vi "Configure Digital Audio Task.vi"(8 "error in (no error)":errorcluster, 11 "digital generation":T2={"data channel list"="", "master clock channel list"="", "digital protocol settings"={"logic level"=enum."3.3 V", "PCM Data Configuration"={"Frame Sync Edge for Channel 0"=enum."Falling", "Channel Count Per Frame"=2, "Channel Length"=32, "Bit Depth"=24, "Channel 0 Offset"=1, "Endianness"=enum."MSB First", "Data Justification"=enum."Left Justified"}, "bit clock rate"=3025000.0, "master clock rate"=3025000.0, "clock mode"=enum."divided clock", "Frame Sync Clock Control"={"Frame Length"=64, "Frame Sync Pulse Width"=32, "Bit Clock Edge  Sync"=enum."Falling"}}, "signal settings"={"signal type"=enum."Sine", "properties"="", "output level units"=enum."% FS"}} {"digital protocol settings"."master clock rate" format="%.4p"; "digital protocol settings"."bit clock rate" format="%.4p"}) -> (0 "error out":errorcluster, 2 "master clock task":T1, 3 "data task":T1)   [LabVIEW 2021, in "DigitalAudioGenerationProcess.lvlib"]
uses:
  DigitalAudioGenerationProcess.lvlib
  controls/digital generation settings.ctl
  controls/digital protocol settings.ctl
  <vilib>/PDM Acquisition Toolkit/host/Classes/Session/Controls/Logic Levels.ctl
  <vilib>/PDM Acquisition Toolkit/shared/controls/PCM Data Format Configuration.ctl
  <vilib>/PDM Acquisition Toolkit/shared/controls/Digital Edge.ctl
  <vilib>/PDM Acquisition Toolkit/shared/controls/PCM Bit Endianness.ctl
  <vilib>/PDM Acquisition Toolkit/shared/controls/PCM Data Justification.ctl
  <vilib>/PDM Acquisition Toolkit/shared/controls/clock mode.ctl
  <vilib>/PDM Acquisition Toolkit/shared/controls/PCM Frame Sync Control.ctl
  controls/signal settings.ctl
  controls/signal type.ctl
  shared/controls/digital output level units.ctl
  <vilib>/PDM Acquisition Toolkit/host/Classes/Tasks/PCM Output/Controls/PCM Output Task DVR.ctl
  <vilib>/PDM Acquisition Toolkit/host/Classes/Tasks/PCM Output/PCM Output Task.lvclass
  controls/sine wave properties.ctl
  <vilib>/PDM Acquisition Toolkit/host/API/Public/Function Generator/Configure Custom Signal (N Ch) - PCM Output Task.vi
  <vilib>/PDM Acquisition Toolkit/shared/PDM Shared.lvlib
  <vilib>/PDM Acquisition Toolkit/host/API/PDM Acquisition Toolkit.lvlib
  controls/AudioGenTypeDefs.lvlib
  <vilib>/PDM Acquisition Toolkit/host/Classes/Session/DecoderSession.lvclass
  shared/controls/audio controls.lvlib
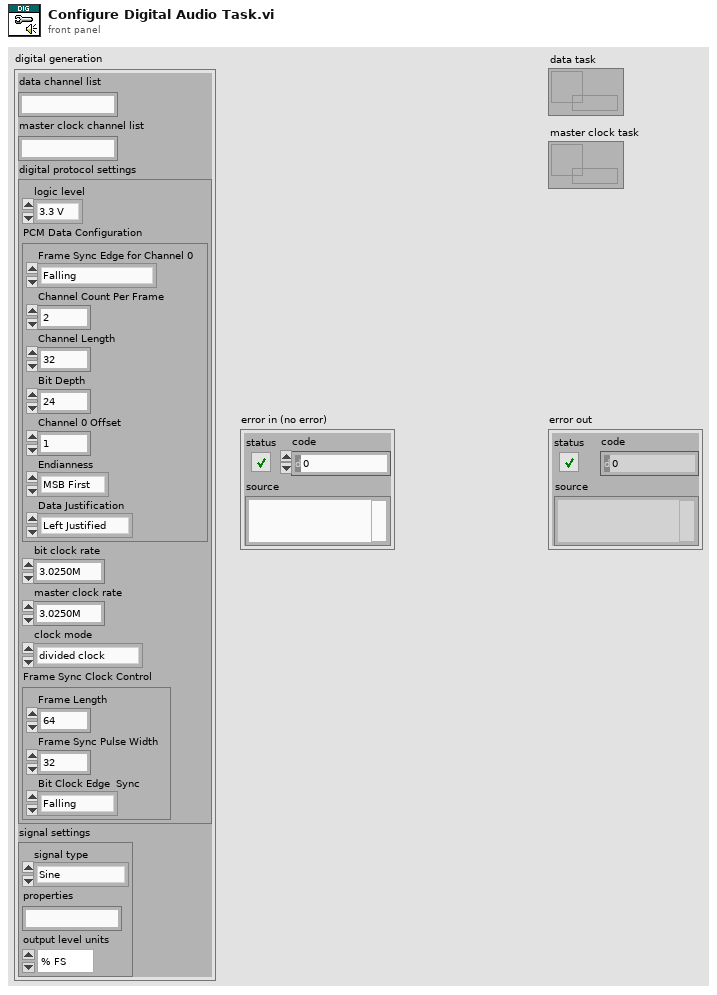
[diagram p1: front panel]
types:
  T1 = typedef "PDM Acquisition Class Library.lvlib/PCM Output Task.lvclass/PCM Output Task DVR.ctl" = refnum<data-value>
  T2 = typedef "AudioGenTypeDefs.lvlib/digital generation settings.ctl" = cluster{"data channel list":string, "master clock channel list":string, "digital protocol settings":T3, "signal settings":T11}
  T3 = typedef "AudioGenTypeDefs.lvlib/digital protocol settings.ctl" = cluster{"logic level":T4, "PCM Data Configuration":T5, "bit clock rate":sgl, "master clock rate":sgl, "clock mode":T9, "Frame Sync Clock Control":T10}
  T4 = typedef "PDM Acquisition Class Library.lvlib/DecoderSession.lvclass/Logic Levels.ctl" = enum16{"3.3 V", "1.8 V", "1.2 V"}
  T5 = typedef "PDM Shared.lvlib/PCM Data Format Configuration.ctl" = cluster{"Frame Sync Edge for Channel 0":T6, "Channel Count Per Frame":u8, "Channel Length":u16, "Bit Depth":u8, "Channel 0 Offset":u16, "Endianness":T7, "Data Justification":T8}
  T6 = typedef "PDM Shared.lvlib/Digital Edge.ctl" = enum8{"Rising", "Falling"}
  T7 = typedef "PDM Shared.lvlib/PCM Bit Endianness.ctl" = enum16{"MSB First", "LSB First"}
  T8 = typedef "PDM Shared.lvlib/PCM Data Justification.ctl" = enum16{"Left Justified", "Right Justified"}
  T9 = typedef "PDM Shared.lvlib/clock mode.ctl" = enum16{"divided clock", "DDS"}
  T10 = typedef "PDM Shared.lvlib/PCM Frame Sync Control.ctl" = cluster{"Frame Length":u16, "Frame Sync Pulse Width":u16, "Bit Clock Edge  Sync":T6}
  T11 = typedef "AudioGenTypeDefs.lvlib/signal settings.ctl" = cluster{"signal type":T12, "properties":string, "output level units":T13}
  T12 = typedef "AudioGenTypeDefs.lvlib/signal type.ctl" = enum16{"Sine", "Dual Tone"}
  T13 = typedef "audio controls.lvlib/digital output level units.ctl" = enum32{"% FS", "dBFS", "V"}
  T14 = typedef "AudioGenTypeDefs.lvlib/sine wave properties.ctl" = cluster{"frequency":dbl, "amplitude":dbl, "phase":dbl}[]
  T15 = typedef "PDM Acquisition Class Library.lvlib/I2S Output Task.lvclass/SignalProperties.ctl" = cluster{"cyclic signal":dbl[], "channel parameters":T16[]}
  T16 = typedef "PDM Acquisition Class Library.lvlib/I2S Output Channel.lvclass/GenerationChannelProperties.ctl" = cluster{"cyclic period":dbl, "cyclic phase offset":dbl, "gain":dbl}
  T17 = typedef "AudioGenTypeDefs.lvlib/dual tone properties.ctl" = cluster{"IMD standard":T18, "low frequency":dbl, "high frequency":dbl, "amplitude ratio":dbl, "ampltidue":dbl}
  T18 = typedef "AudioGenTypeDefs.lvlib/dual tone types.ctl" = enum32{"SMPTE 4:1", "DIN", "CCIF 11k-12k", "CCIF 19k-20k", "Custom"}
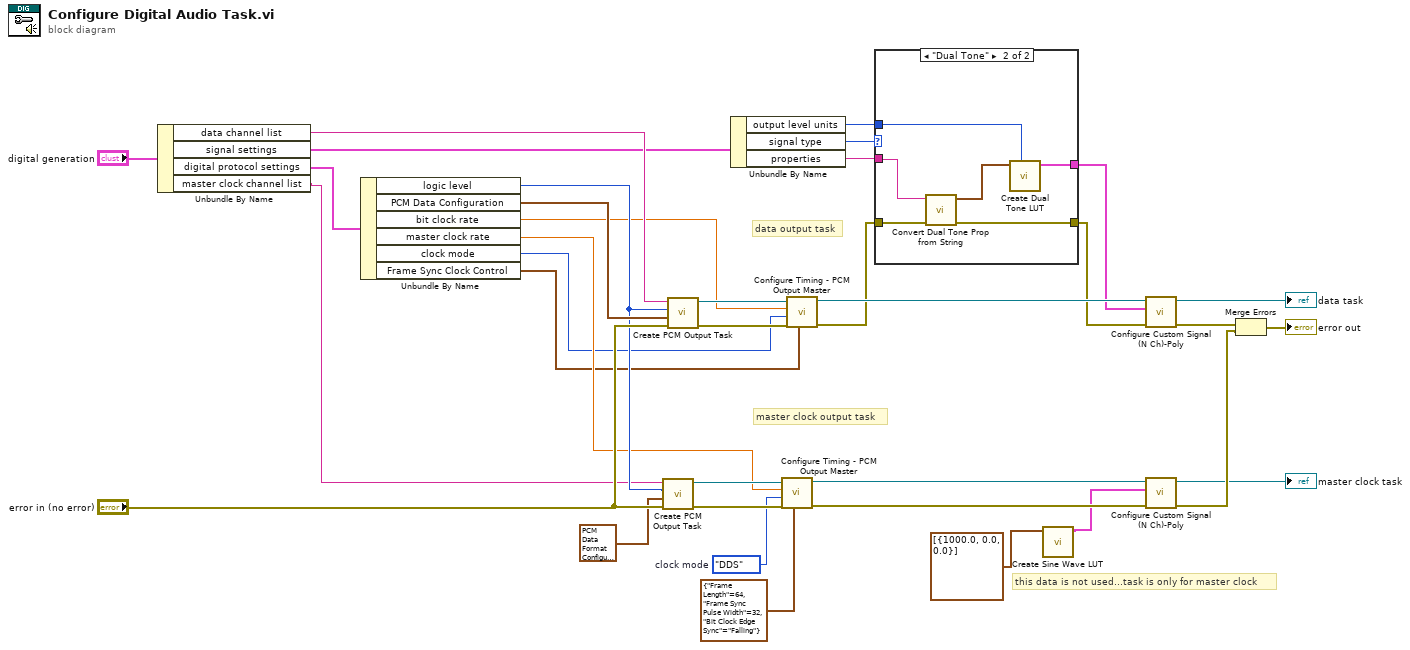
[diagram p0: block diagram]
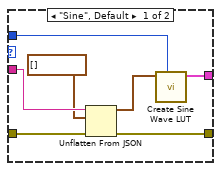
[diagram p2: hidden frame]
diagram:
  w31 = clock_mode."DDS"  # clock mode
  # "this data is not used...task is only for master clock"
  # "master clock output task"
  # "data output task"
  n1 = Unbundle By Name("digital generation") -> ("data channel list"=w21:string, "signal settings"=w6:T11, "digital protocol settings"=w20:T3, "master clock channel list"=w12:string)
  n2 = Unbundle By Name(w20) -> ("logic level"=w17:T4, "PCM Data Configuration"=w19:T5, "bit clock rate"=w16:sgl, "master clock rate"=w15:sgl, "clock mode"=w14:T9, "Frame Sync Clock Control"=w13:T10)
  n3 = call <vilib>:"Create PCM Output Task.vi"("error in"="error in (no error)", "PCM data configuration"=T5 {"Frame Sync Edge for Channel 0"=enum."Falling", "Channel Count Per Frame"=2, "Channel Length"=32, "Bit Depth"=24, "Channel 0 Offset"=1, "Endianness"=enum."MSB First", "Data Justification"=enum."Left Justified"} ("PCM Data Configuration 2"), "logic level"=w17, "channel list"=w12) -> ("error out"=w32:errorcluster, "PCM output task out"=w33:T1)  [unwired: 6 in]
  n4 = call <vilib>:"Create PCM Output Task.vi"("error in"="error in (no error)", "PCM data configuration"=w19, "logic level"=w17, "channel list"=w21) -> ("error out"=w34:errorcluster, "PCM output task out"=w35:T1)  [unwired: 6 in]
  n5 = Unbundle By Name(w6) -> ("output level units"=w1:T13, "signal type"=w5:T12, "properties"=w4:string)
  n6 = call <vilib>:"Configure Timing - PCM Output Master.vi"("Frame Sync Clock Control"=T10 {"Frame Length"=64, "Frame Sync Pulse Width"=32, "Bit Clock Edge  Sync"=enum."Falling"} ("Frame Sync Clock Control 2"), "error in"=w32, "clock mode"=w31, "Bit Clock rate"=w15, "PCM output task in"=w33) -> ("error out"=w29:errorcluster, "PCM output task out"=w28:T1)  [unwired: 4 in, 1 out]
  n7 = call <vilib>:"Configure Timing - PCM Output Master.vi"("Frame Sync Clock Control"=w13, "error in"=w34, "clock mode"=w14, "Bit Clock rate"=w16, "PCM output task in"=w35) -> ("error out"=w8:errorcluster, "PCM output task out"=w27:T1)  [unwired: 4 in, 1 out]
  n8 = case shown="\"Dual Tone\"" w5 {
    tunnel: [w42 w45] -> w9
    tunnel: w8 -> [w41 w48]
    tunnel: [w40 w47] -> w7
    tunnel: w4 -> [w39 w46]
    tunnel: w1 -> [w36 w44]
    frame "Sine", Default {
      n9 = Unflatten From JSON(JSON string=w39, type and defaults=T14 [] ("sine wave properties"), error in (no error)=w41) -> (value=w37:T14, error out=w40:errorcluster)  [unwired: 4 in]
      n10 = call "Create Sine Wave LUT.vi"("output level units"=w36, "sine wave properties"=w37) -> ("Signal Properties"=w42:T15)  [unwired: 9 in]
    }
    frame "Dual Tone" {
      n11 = call "Convert Dual Tone Prop from String.vi"("error in (no error)"=w48, "dual tone properties"=w46) -> ("error out"=w47:errorcluster, "dual tone properties"=w43:T17)  [unwired: 8 in]
      n12 = call "Create Dual Tone LUT.vi"("output level units"=w44, "dual tone properties"=w43) -> ("Signal Properties"=w45:T15)  [unwired: 9 in]
    }
  }
  n13 = call "Create Sine Wave LUT.vi"("sine wave properties"=T14 [{"frequency"=1000.0, "amplitude"=0.0, "phase"=0.0}]) -> ("Signal Properties"=w3:T15)  [unwired: 10 in]
  n14 = call-poly <vilib>:"Configure Custom Signal (N Ch)-Poly.vi"("error in"=w7, "signal parameters"=w9, "PCM output task in"=w27) -> ("error out"=w25:errorcluster, "PCM output task out"=→"data task":T1)  [unwired: 7 in]
  n15 = call-poly <vilib>:"Configure Custom Signal (N Ch)-Poly.vi"("error in"=w29, "signal parameters"=w3, "PCM output task in"=w28) -> ("error out"=w24:errorcluster, "PCM output task out"=→"master clock task":T1)  [unwired: 7 in]
  n16 = Merge Errors(w25, w24) -> (→"error out":errorcluster)
